vi "RoiSelectionArrayCalcAndor1.vi"(0 "Zoom in":bool, 1 "Index In":i32 min=0 max=2, 5 "Zoom out":bool, 7 "IntensityGraphAndor0_Display":i32[][](graph), 9 "ROI Square in":bool, 11 "error in (no error)":errorcluster) -> (3 "Image Out":T1(plugin-control), 4 "Intensity Graph Out":i32[][](graph), 6 "ROI Intensity Graph Out":i32[][](graph), 15 "error out":errorcluster)   [LabVIEW 2011]
uses:
  <vilib>/Utility/inputDevices.llb/mouseAcquire.vi
panel:
  out "Zoom-Faktor":dbl
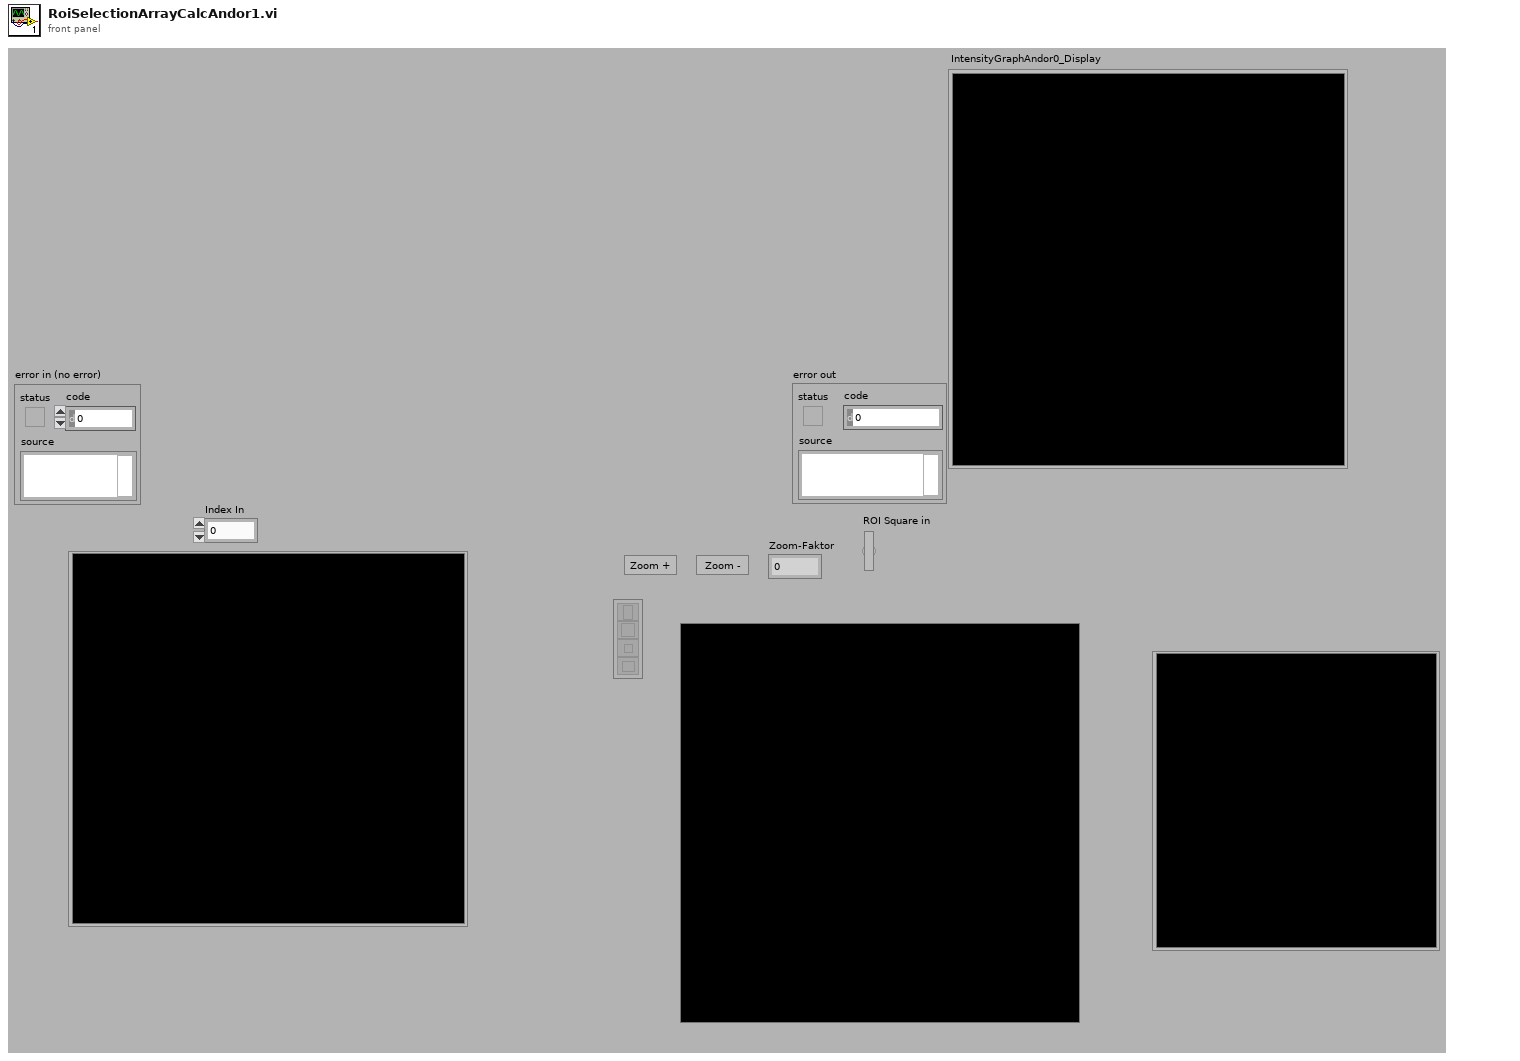
[diagram p1: front panel]
types:
  T1 = typedef "IMAQ Image.ctl" = refnum<image>
  T2 = cluster{"Left":i32, "Top":i32, "Right":i32, "Bottom":i32}
  T3 = cluster{"button 1":bool, "button 2":bool, "button 3":bool, "button 4":bool}
  T4 = cluster{"Global Rectangle":i32[], "Contours":cluster{"Contour Type":u32, "ROI Type":u32, "Points":i32[]}[]}
  T5 = cluster{"Contour Type":u32, "ROI Type":u32, "Points":i32[]}[]
  T6 = cluster{"Contour Type":u32, "ROI Type":u32, "Points":i32[]}
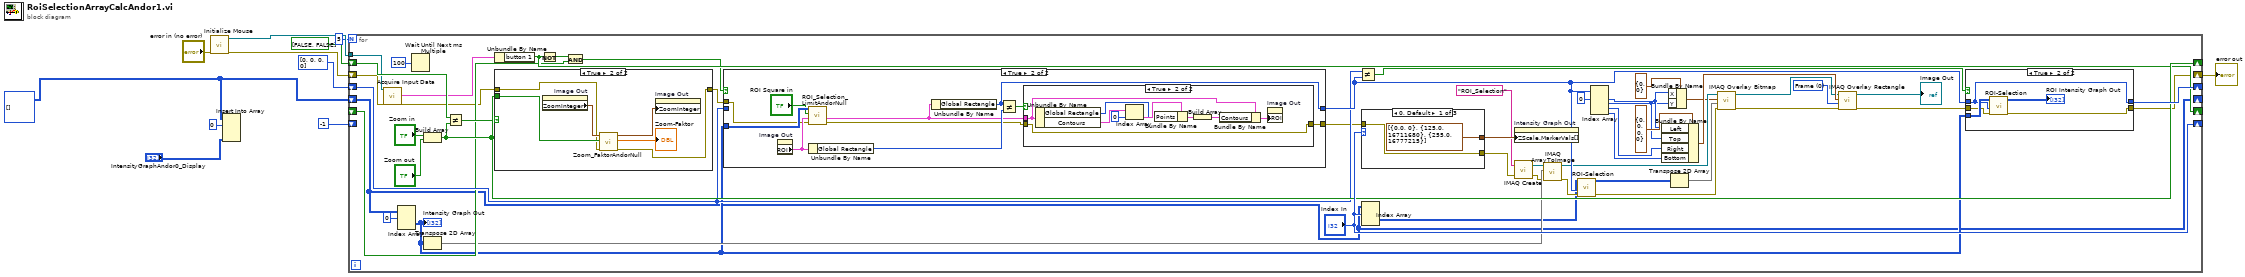
[diagram p0: block diagram]
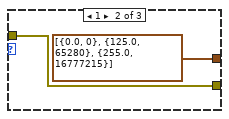
[diagram p2: hidden frame]
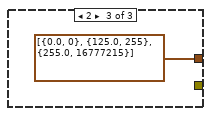
[diagram p3: hidden frame]
diagram:
  w3 = i32[][][] []
  n1 = call <vilib>:"Initialize Mouse.vi"("error in (no error)"="error in (no error)") -> ("error out"=w7:errorcluster, "device ID"=w8:refnum<k1>)  [unwired: 9 in]
  n2 = Insert Into Array(array=w3, index (dim 0)=0 ("index (page)"), new element="IntensityGraphAndor0_Display") -> ()  [unwired: 2 in, 1 out]
  n3 = for {
    N: 5 -> [_]
    shift-right: ["Index In"] -> _
    shift-left: -1 ("index (page)") -> [_]
    shift-right: [w61] -> _
    shift-left: i32[] [0, 0, 0, 0] ("Global Rectangle") -> [w52]
    shift-right: [w56] -> _
    shift-left: bool[] [FALSE, FALSE] -> [w57]
    tunnel: w8 -> [w51]
    shift-right: [w49] -> _
    shift-left: _ -> [w47]
    shift-right: [w16] -> w5
    shift-left: w7 -> [w15]
    shift-right: [w12] -> _
    shift-left: w3 -> [w12]
    w34 = u32 0 items=["Frame", "Fill", "Highlight"] ("Drawing Mode (Frame)")
    n4 = call-poly <vilib>:"Acquire Input Data.vi"("device ID"=w51, "error in (no error)"=w15) -> ("button info"=w50:T3, "error out"=w37:errorcluster)  [unwired: 14 in, 2 out]
    n5 = Index Array(array=w12, index (dim 0)=0 ("index (page)")) -> (element=w14:i32[][])  [unwired: 2 in]
    "Intensity Graph Out" <- w14
    n6 = Wait Until Next ms Multiple(millisecond multiple=u32 100) -> ()  [unwired: 1 out]
    n7 = Build Array("Zoom in", "Zoom out") -> (w56:bool[])
    n8 = Transpose 2D Array(2D array=w14) -> (transposed array=w42:i32[][])
    n9 = Not Equal?(x=w57, y=w56) -> (x != y?=w55:bool)
    n10 = Unbundle By Name(w50) -> ("button 1"=w49:bool)
    n11 = case shown="True" w55 {
      tunnel: w56 -> [_ w94]
      tunnel: w37 -> [w90 w92]
      tunnel: [w90 w91] -> w19
      frame False {
      }
      frame True {
        n12 = property on="Image Out" class="ImageControl"() -> ("ZoomInteger"=w95:cluster{"X":i32, "Y":i32})  [unwired: 2 in, 2 out]
        n13 = call "Zoom_FaktorAndorNull.vi"("error in (no error)"=w92, "Array"=w94, "ZoomInteger 2"=w95) -> ("error out"=w91:errorcluster, "X"=→"Zoom-Faktor":dbl, "ZoomInteger"=w93:cluster{"X":i32, "Y":i32})  [unwired: 6 in]
        n14 = property on="Image Out" class="ImageControl"("ZoomInteger"=w93) -> ()  [unwired: 2 in, 2 out]
      }
    }
    n15 = Not(x=w49) -> (.not. x?=w48:bool)
    n16 = And(x=w48, y=w47) -> (x .and. y?=w46:bool)
    n17 = case shown="True" w46 {
      tunnel: w14 -> [_ w79]
      tunnel: [w69 w77] -> w53
      tunnel: w52 -> [w69 _]
      tunnel: w19 -> [w68 w72]
      tunnel: [w68 w70] -> w18
      frame False {
      }
      frame True {
        n18 = property on="Image Out" class="ImageControl"() -> ("ROI"=w78:T4)  [unwired: 2 in, 2 out]
        n19 = call "ROI_Selection_LimitAndorNull.vi"("error in (no error)"=w72, "ROI in"=w78, "Square"="ROI Square in", "Picture"=w79) -> ("error out"=w71:errorcluster, "ROI out"=w75:T4)  [unwired: 6 in]
        n20 = Unbundle By Name(w78) -> ("Global Rectangle"=w76:i32[])
        n21 = Unbundle By Name(w75) -> ("Global Rectangle"=w77:i32[])
        n22 = Not Equal?(x=w77, y=w76) -> (x != y?=w74:bool)
        n23 = case shown="True" w74 {
          tunnel: w75 -> [_ w84]
          tunnel: w71 -> [w80 w81]
          tunnel: [w80 w81] -> w70
          frame False {
          }
          frame True {
            n24 = Unbundle By Name(w84) -> ("Global Rectangle"=w86:i32[], "Contours"=w88:T5)
            n25 = Index Array(array=w88, index=0) -> (element=w87:T6)
            n26 = Bundle By Name(cluster=w87, "Points"=w86) -> (w85:T6)
            n27 = Build Array(w85) -> (w83:T5)
            n28 = Bundle By Name(cluster=w84, "Contours"=w83) -> (w82:T4)
            n29 = property on="Image Out" class="ImageControl"("ROI"=w82) -> ()  [unwired: 2 in, 2 out]
          }
        }
      }
    }
    n30 = Not Equal?(x=w52, y=w53) -> (x != y?=w54:bool)
    n31 = case shown="0, Default" "Index In" {
      tunnel: [cluster{dbl, u32}[] [{0.0, 0}, {125.0, 16711680}, {255.0, 16777215}] ("Z Scale.Marker Values[]") cluster{dbl, u32}[] [{0.0, 0}, {125.0, 65280}, {255.0, 16777215}] ("Z Scale.Marker Values[]") cluster{dbl, u32}[] [{0.0, 0}, {125.0, 255}, {255.0, 16777215}] ("Z Scale.Marker Values[]")] -> w44
      tunnel: w18 -> [w63 w65 _]
      tunnel: [w63 w65 _] -> w17
      frame 0, Default {
      }
      frame 1 {
      }
      frame 2 {
      }
    }
    n32 = Index Array(array=w12, index (dim 0)="Index In") -> (element=w13:i32[][])  [unwired: 2 in]
    n33 = property on="Intensity Graph Out" class="IntGraph (strict)"("ZScale.MarkerVals[]"=w44) -> ()  [unwired: 2 in, 2 out]
    n34 = call "IMAQ Create"("Image Name"="ROI_Selection", "error in (no error)"=w17) -> ("New Image"=w43:T1, "error out"=w41:errorcluster)  [unwired: 3 in]
    n35 = call "IMAQ ArrayToImage"("error in (no error)"=w41, "Image Pixels (U8)"=w42, "Image"=w43) -> ("error out"=w22:errorcluster, "Image Out"=w39:T1)  [unwired: 7 in]
    n36 = call "ROI-Selection.vi"("error in (no error)"=w22, "Global Rectangle"=w53, "Image In"=w13) -> ("error out"=w21:errorcluster, "Image Out"=w23:i32[][])  [unwired: 7 in]
    n37 = Index Array(array=w53, index #1=0 ("index")) -> (element #1=w30:i32, element #2=w29:i32, element #3=w32:i32, element #4=w31:i32)  [unwired: 3 in]
    n38 = Bundle By Name(cluster=T2 {"Left"=0, "Top"=0, "Right"=0, "Bottom"=0} ("Rectangle"), "Left"=w30, "Top"=w29, "Right"=w32, "Bottom"=w31) -> (w33:T2)
    n39 = Bundle By Name(cluster=cluster{"X":i32, "Y":i32} {"X"=0, "Y"=0} ("Top Left Point"), "X"=w30, "Y"=w29) -> (w25:cluster{"X":i32, "Y":i32})
    n40 = Transpose 2D Array(2D array=w23) -> (transposed array=w24:i32[][])
    n41 = call "IMAQ Overlay Bitmap"("error in (no error)"=w21, "Bitmap"=w24, "Top Left Point"=w25, "Image"=w39) -> ("error out"=w27:errorcluster, "Image Out"=w28:T1)  [unwired: 6 in]
    n42 = call "IMAQ Overlay Rectangle"("error in (no error)"=w27, "Drawing Mode (Frame)"=w34, "Rectangle"=w33, "Image"=w28) -> ("error out"=w20:errorcluster, "Image Out"=→"Image Out":T1)  [unwired: 6 in]
    n43 = case shown="True" w54 {
      tunnel: w14 -> [_ w103]
      tunnel: w53 -> [w98 w102]
      tunnel: [w98 w102] -> w61
      tunnel: w20 -> [w97 w100]
      tunnel: [w97 w99] -> w16
      frame False {
      }
      frame True {
        n44 = call "ROI-Selection.vi"("error in (no error)"=w100, "Global Rectangle"=w102, "Image In"=w103) -> ("error out"=w99:errorcluster, "Image Out"=→"ROI Intensity Graph Out":i32[][])  [unwired: 7 in]
      }
    }
  }
  "error out" <- w5
